vi "Run_Display.vi"(4 "Numeric":u32) -> (1 "Colors [4]":cluster{u32, u32}[](array[cluster]))   [LabVIEW 2019]
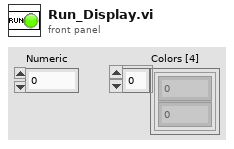
[diagram p1: front panel]
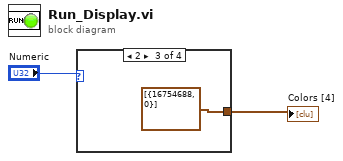
[diagram p0: block diagram]
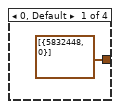
[diagram p2: hidden frame]
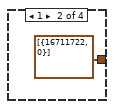
[diagram p3: hidden frame]
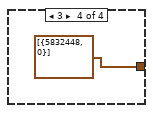
[diagram p4: hidden frame]
diagram:
  n1 = case shown="2" "Numeric" {
    tunnel: [cluster{u32, u32}[] [{5832448, 0}] ("Colors [4]") cluster{u32, u32}[] [{16711722, 0}] ("Colors [4]") cluster{u32, u32}[] [{16754688, 0}] ("Colors [4]") cluster{u32, u32}[] [{5832448, 0}] ("Colors [4]")] -> w2
    frame 0, Default {
    }
    frame 1 {
    }
    frame 2 {
    }
    frame 3 {
    }
  }
  "Colors [4]" <- w2
